vi "ReadPositionRegister.vi"(0 "error in":errorcluster, 5 "Snpx":refnum<k24>, 11 "index":i32) -> (4 "error out":errorcluster, 6 "UserFrame":i16, 8 "Cartesian position":T1, 10 "UserTool":i16, 15 "Joint position":dbl[](array[numeric]))   [LabVIEW 2010, in "UnderAutomation.Fanuc.lvlib"]
uses:
  UnderAutomation.Fanuc.lvlib
  C:/Users/fg/Documents/Fanuc.vi/LabVIEW_2024/UnderAutomation.Fanuc/lib/UnderAutomation.Fanuc.dll
  LabVIEW_2024/UnderAutomation.Fanuc/lib/UnderAutomation.Fanuc.dll
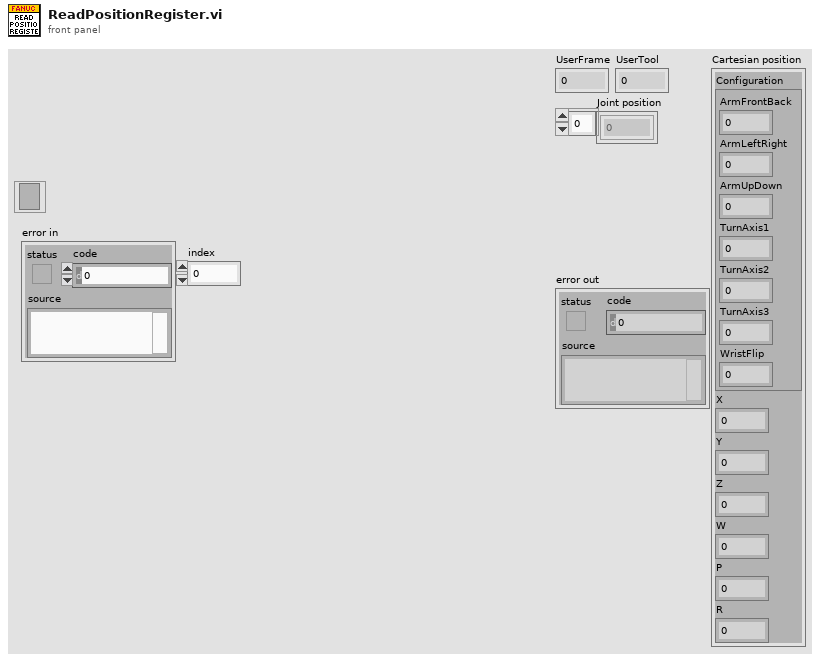
[diagram p1: front panel]
types:
  T1 = cluster{"Configuration":cluster{"ArmFrontBack":i32, "ArmLeftRight":i32, "ArmUpDown":i32, "TurnAxis1":i32, "TurnAxis2":i32, "TurnAxis3":i32, "WristFlip":i32}, "X":dbl, "Y":dbl, "Z":dbl, "W":dbl, "P":dbl, "R":dbl}
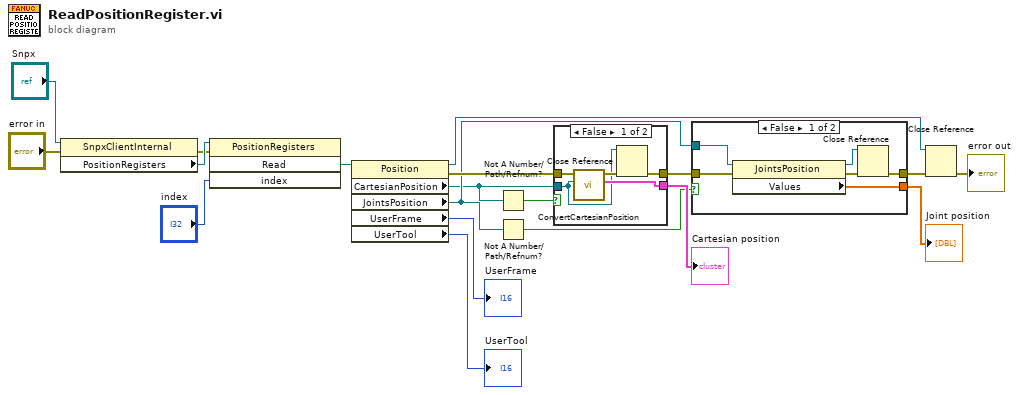
[diagram p0: block diagram]
diagram:
  n1 = property class="SnpxClientInternal"(reference="Snpx", error in="error in") -> (error out=w16:errorcluster, "PositionRegisters"=w17:refnum<k24>)  [unwired: 1 out]
  n2 = invoke class="PositionRegisters" method="Read"(reference=w17, error in=w16, "index"="index") -> ("Read"=w14:refnum<k24>)  [unwired: 1 in, 3 out]
  n3 = property class="Position"(reference=w14) -> (reference out=w1:refnum<k24>, error out=w10:errorcluster, "CartesianPosition"=w2:refnum<k24>, "JointsPosition"=w8:refnum<k24>, "UserFrame"=→"UserFrame":i16, "UserTool"=→"UserTool":i16)  [unwired: 1 in]
  n4 = Not A Number/Path/Refnum?(number/path/refnum=w2) -> (NaN/Path/Refnum?=w11:bool)
  n5 = Not A Number/Path/Refnum?(number/path/refnum=w8) -> (NaN/Path/Refnum?=w7:bool)
  n6 = case shown="False" w11 {
    tunnel: w2 -> [w20 _]
    tunnel: w10 -> [w24 w25]
    tunnel: [w23 _] -> w9
    tunnel: [w21 w25] -> w5
    frame False {
      n7 = call "ConvertCartesianPosition.vi"("Cartesian position"=w20, "error in (no error)"=w24) -> ("Cartesian position"=w23:T1, "error out"=w22:errorcluster)  [unwired: 8 in]
      n8 = Close Reference(reference=w20, error in (no error)=w22) -> (error out=w21:errorcluster)
    }
    frame True {
    }
  }
  "Cartesian position" <- w9
  n9 = case shown="False" w7 {
    tunnel: w8 -> [w31 _]
    tunnel: [w30 _] -> w6
    tunnel: w5 -> [w29 w32]
    tunnel: [w26 w32] -> w4
    frame False {
      n10 = property class="JointsPosition"(reference=w31, error in=w29) -> (reference out=w28:refnum<k24>, error out=w27:errorcluster, "Values"=w30:dbl[])
      n11 = Close Reference(reference=w28, error in (no error)=w27) -> (error out=w26:errorcluster)
    }
    frame True {
    }
  }
  "Joint position" <- w6
  n12 = Close Reference(reference=w1, error in (no error)=w4) -> (error out=→"error out":errorcluster)
